vi "Test Panel.vi"(8 "error in (no error)":errorcluster, 11 "Node Ptr":T2 format="%.0x") -> (0 "error out":errorcluster)   [LabVIEW 2019]
uses:
  <vilib>/NI VeriStand/Custom Device API/Custom Device Item Ref.ctl
  <vilib>/NI VeriStand/UI Controls/Tree and Alias Browser/Tree Alias Browser Display.ctl
  NationalInstruments.VeriStand.SystemDefinitionAPI
  NationalInstruments.VeriStand.SystemStorage
  <vilib>/NI VeriStand/Custom Device API/Custom Device API.lvlib
  <vilib>/NI VeriStand/UI Controls/Tree and Alias Browser/NI_VS UI Tree Alias Browser.lvlib
  Software Multi-Plex System Explorer.lvlib
  NationalInstruments.VeriStand.SystemStorageUI
panel:
  in  "error in (no error) 2":errorcluster
  in  "System Definition":path
  in  "Map Input":bool
  out "Input Path":string
  in  "Tree Browser":T1
  in  "Specific Header":cluster{"Section Name":string}={"Section Name"="Specify Input 1 Channel Source"}
  in  "General Header":cluster{"Section Name":string}={"Section Name"="Software Multi-Plex Channel Input 1 Settings"}
  in  "Description":string
  in  "Name":string
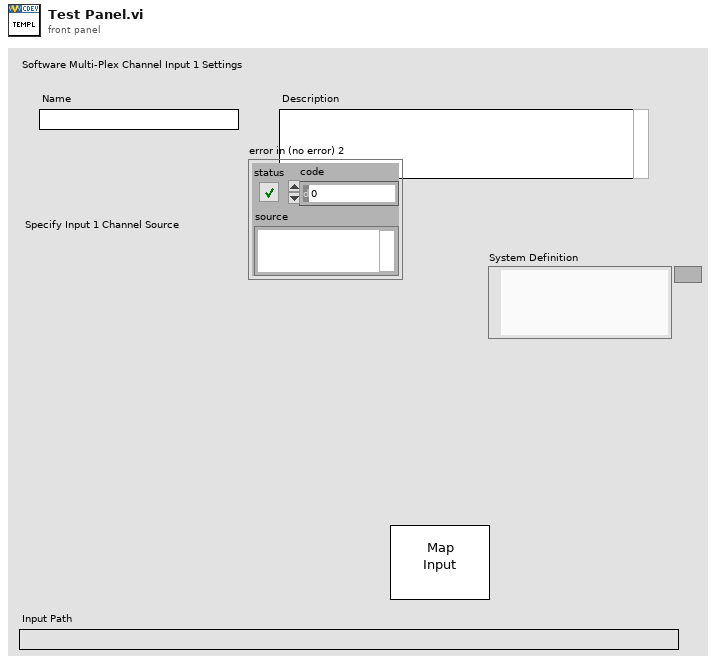
[diagram p1: front panel]
types:
  T1 = typedef "NI_VS UI Tree Alias Browser.lvlib/Tree Alias Browser Display.ctl" = refnum<k24>
  T2 = typedef "Custom Device API.lvlib/Custom Device Item Ref.ctl" = u64
  T3 = typedef "Custom Device API.lvlib/Custom Device Item Info.ctl" = cluster{"Name":string, "Is Channel":bool, "GUID":string, "Is Waveform":bool}
  T4 = typedef "NI_VS UI Tree Alias Browser.lvlib/Callback Type.ctl" = cluster{"Net Callbacks":refnum<k27>[], "Event":T5}
  T5 = typedef "NI_VS UI Tree Alias Browser.lvlib/Net Event Data Ref.ctl" = refnum<user-event>
  T6 = typedef "NI_VS UI Tree Alias Browser.lvlib/Tree Alias Browser Ref.ctl" = refnum<k24>
  T7 = typedef "Custom Device API.lvlib/Custom Device Commands.ctl" = enum16{"Default", "Item renamed", "Shutdown", "Dynamic button pressed"}
  T8 = typedef "NI_VS UI Tree Alias Browser.lvlib/Net Event.ctl" = enum16{"SelectedItem", "DblClick"}
  T9 = typedef "Custom Device API.lvlib/Custom Device Pointer.ctl" = refnum<k24>
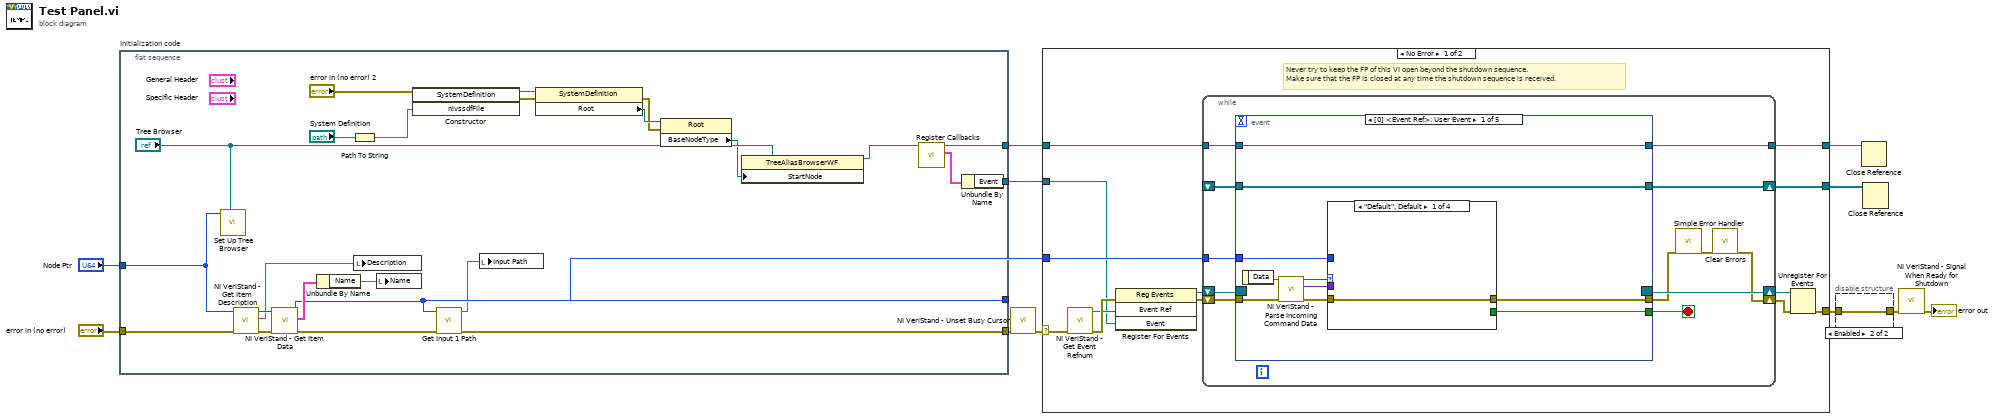
[diagram p0: block diagram]
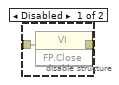
[diagram p2: hidden frame]
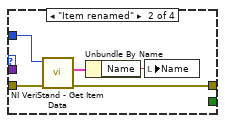
[diagram p3: hidden frame]
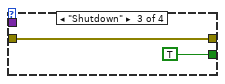
[diagram p4: hidden frame]
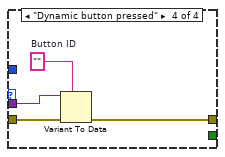
[diagram p5: hidden frame]
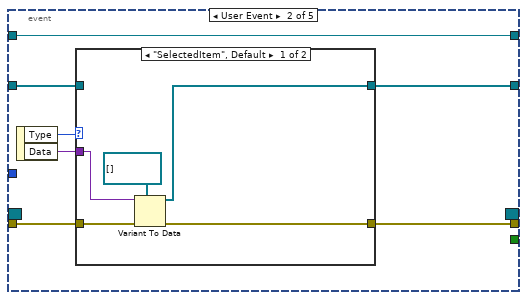
[diagram p6: hidden frame]
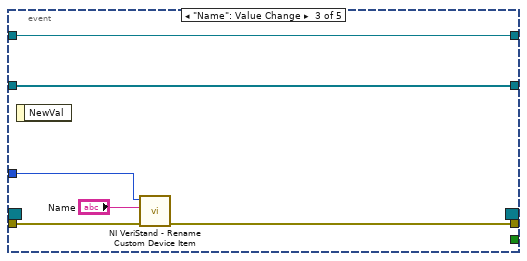
[diagram p8: hidden frame]
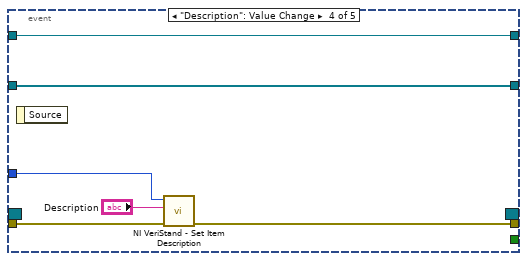
[diagram p9: hidden frame]
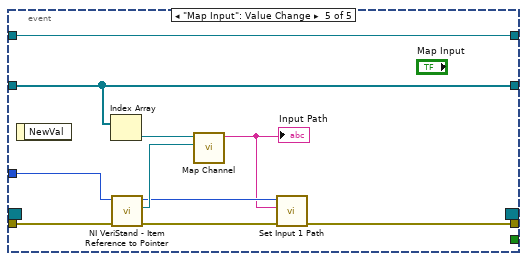
[diagram p10: hidden frame]
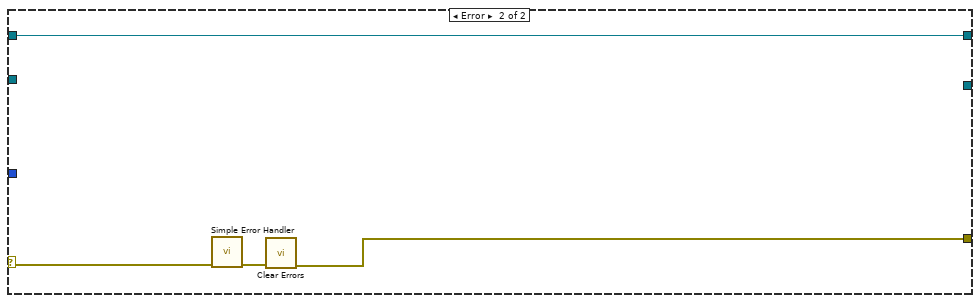
[diagram p11: hidden frame]
diagram:
  n1 = flat-sequence "Initialization code" {
    tunnel: "error in (no error)" -> [w31]
    tunnel: "Node Ptr" -> [w30]
    tunnel: [w25] -> w8
    tunnel: [w24] -> w5
    tunnel: [w29] -> w4
    tunnel: [w27] -> w2
    frame #0 {
      n2 = call "Set Up Tree Browser.vi"("Tree Ref"="Tree Browser", "Item Ref in"=w30) -> ()  [unwired: 10 in]
      n3 = call <vilib>:"NI VeriStand - Get Item Description.vi"("error in (no error)"=w31, "Item Ref in"=w30) -> ("error out"=w35:errorcluster, "Description"=w32:string, "Item Ref out"=w36:T2)  [unwired: 7 out]
      n4 = call <vilib>:"NI VeriStand - Get Item Data.vi"("error in (no error)"=w35, "Item Ref in"=w36) -> ("error out"=w26:errorcluster, "Item Info"=w34:T3, "Item Ref out"=w24:T2)  [unwired: 7 out]
      n5 = Unbundle By Name(w34) -> ("Name"=w33:string)
      n6 = Path To String(path="System Definition") -> (string=w16:string)
      n7 = local write "Description"(w32) -> ()
      n8 = local write "Name"(w33) -> ()
      n9 = constructor class="SystemDefinition"(error in="error in (no error) 2", "nivssdfFile"=w16) -> (reference out=w21:refnum<k24>, error out=w20:errorcluster)  [unwired: 2 in, 2 out]
      n10 = call "Get Input 1 Path.vi"("error in (no error)"=w26, "Item Ref in"=w24) -> ("error out"=w25:errorcluster, "Input Path"=w23:string)  [unwired: 8 in]
      n11 = local write "Input Path"(w23) -> ()
      n12 = property class="SystemDefinition"(reference=w21, error in=w20) -> (error out=w18:errorcluster, "Root"=w19:refnum<k24>)  [unwired: 1 out]
      n13 = property class="Root"(reference=w19, error in=w18) -> ("BaseNodeType"=w13:refnum<k24>)  [unwired: 2 out]
      n14 = property class="TreeAliasBrowserWF"(reference="Tree Browser", "StartNode"=w13) -> (reference out=w14:T1)  [unwired: 1 in, 1 out]
      n15 = call <vilib>:"Register Callbacks.vi"("Tree Alias"=w14) -> ("Callbacks"=w28:T4, "Tree Alias dup"=w29:T6)  [unwired: 8 in, 1 out]
      n16 = Unbundle By Name(w28) -> ("Event"=w27:T5)
    }
  }
  n17 = call <vilib>:"NI VeriStand - Unset Busy Cursor.vi"("error in (no error)"=w8) -> ("error out"=w7:errorcluster)  [unwired: 10 out]
  n18 = case shown="No Error" w7 {
    selector: w7 -> [w41 w123]
    tunnel: [w46 w121] -> w12
    tunnel: w5 -> [w42 _]
    tunnel: w4 -> [w40 w120]
    tunnel: [w39 w120] -> w3
    tunnel: w2 -> [w38 _]
    tunnel: [w37 _] -> w1
    frame No Error {
      # "Never try to keep the FP of this VI open beyond the shutdown sequence.\nMake sure that the FP is closed at any time the shutdown sequence is received."
      n19 = call <vilib>:"NI VeriStand - Get Event Refnum.vi"("error in (no error)"=w41) -> ("error out"=w49:errorcluster, "Event Ref"=w45:refnum<user-event>)  [unwired: 9 out]
      n20 = register-events(error in=w49, w45, w38) -> (reference out=w43:refnum<event-registration>, error out=w44:errorcluster)  [unwired: 1 in]
      n21 = while {
        tunnel: w42 -> [w57]
        shift-right: [w54] -> w47
        shift-left: w44 -> [w60]
        shift-right: [w61] -> w48
        shift-left: w43 -> [w59]
        tunnel: w40 -> [w53]
        tunnel: [w52] -> w39
        shift-right: [w51] -> w37
        shift-left: _ -> [w50]
        stop <- w58 stop-if-true
        n22 = event shown="[0] <Event Ref>: User Event" {
          selector: w59 -> [_ _ _ _ _]
          dyn-events: [_ _ _ _ _] -> w61
          timeout: _ -> [_ _ _ _ _]
          tunnel: w60 -> [w71 w88 w103 w108 w116]
          tunnel: [w67 _ _ _ _] -> w58
          tunnel: [w66 w87 w102 w107 w110] -> w56
          tunnel: w57 -> [w65 _ w101 w109 w115]
          tunnel: w53 -> [w63 w84 w99 w105 w119]
          tunnel: [w63 w84 w99 w105 w119] -> w52
          tunnel: [w62 w86 w98 w104 w118] -> w51
          tunnel: w50 -> [w62 w85 w98 w104 w118]
          event User Event {
            n23 = event-data() -> ("Data"=w70:string)  [unwired: 1 out]
            n24 = call <vilib>:"NI VeriStand - Parse Incoming Command Data.vi"("error in (no error)"=w71, "Incoming data"=w70) -> ("error out"=w69:errorcluster, "Outgoing data"=w64:variant, "Action"=w68:T7)  [unwired: 7 out]
            n25 = case shown="\"Default\", Default" w68 {
              tunnel: w69 -> [w72 w77 w78 w83]
              tunnel: [_ _ TRUE _] -> w67
              tunnel: [w72 w74 w78 w80] -> w66
              tunnel: w65 -> [_ w76 _ _]
              tunnel: w64 -> [_ _ _ w82]
              frame "Default", Default {
              }
              frame "Item renamed" {
                n26 = call <vilib>:"NI VeriStand - Get Item Data.vi"("error in (no error)"=w77, "Item Ref in"=w76) -> ("error out"=w74:errorcluster, "Item Info"=w75:T3)  [unwired: 8 out]
                n27 = Unbundle By Name(w75) -> ("Name"=w73:string)
                n28 = local write "Name"(w73) -> ()
              }
              frame "Shutdown" {
              }
              frame "Dynamic button pressed" {
                w81 = ""  # Button ID
                n29 = Variant To Data(error in=w83, type=w81, Variant=w82) -> (error out=w80:errorcluster)  [unwired: 1 out]
              }
            }
          }
          event User Event {
            n30 = event-data() -> ("Type"=w90:T8, "Data"=w89:variant)  [unwired: 1 out]
            n31 = case shown="\"SelectedItem\", Default" w90 {
              tunnel: w89 -> [w94 _]
              tunnel: w88 -> [w95 w96]
              tunnel: [w92 w96] -> w87
              tunnel: [w91 w97] -> w86
              tunnel: w85 -> [_ w97]
              frame "SelectedItem", Default {
                n32 = Variant To Data(error in=w95, type=refnum<k24>[] [], Variant=w94) -> (data=w91:refnum<k24>[], error out=w92:errorcluster)
              }
              frame "DblClick" {
              }
            }
          }
          event "Name": Value Change {
            n33 = event-data() -> ()  [unwired: 2 out]
            n34 = call <vilib>:"NI VeriStand - Rename Custom Device Item.vi"("error in (no error)"=w103, "New Name"="Name", "Item Ref in"=w101) -> ("error out"=w102:errorcluster)  [unwired: 1 in, 7 out]
          }
          event "Description": Value Change {
            n35 = event-data() -> ()  [unwired: 2 out]
            n36 = call <vilib>:"NI VeriStand - Set Item Description.vi"("error in (no error)"=w108, "Description"="Description", "Item Ref in"=w109) -> ("error out"=w107:errorcluster)  [unwired: 8 out]
          }
          event "Map Input": Value Change {
            n37 = event-data() -> ()  [unwired: 2 out]
            n38 = Index Array(array=w118) -> (element=w117:refnum<k24>)  [unwired: 1 in]
            n39 = call <vilib>:"NI VeriStand - Item Reference to Pointer.vi"("error in (no error)"=w116, "Item Ref in"=w115) -> ("error out"=w113:errorcluster, "Node Pointer"=w114:T9, "Item Ref out"=w112:T2)  [unwired: 6 in, 1 out]
            n40 = call "Map Channel.vi"("Destination"=w114, "Source"=w117) -> ("Source Path"=w111:string)  [unwired: 8 in, 1 out]
            "Input Path" <- w111
            n41 = call "Set Input 1 Path.vi"("error in (no error)"=w113, "Input Path"=w111, "Item Ref in"=w112) -> ("error out"=w110:errorcluster)  [unwired: 8 in]
          }
        }
        n42 = call <vilib>:"Simple Error Handler.vi"("error in (no error)"=w56) -> ("error out"=w55:errorcluster)  [unwired: 1 in, 7 out]
        n43 = call <vilib>:"Clear Errors.vi"("error in (no error)"=w55) -> ("error out"=w54:errorcluster)  [unwired: 1 in, 5 out]
      }
      n44 = Unregister For Events(event registration refnum=w48, error in=w47) -> (error out=w46:errorcluster)
    }
    frame Error {
      n45 = call <vilib>:"Simple Error Handler.vi"("error in (no error)"=w123) -> ("error out"=w122:errorcluster)  [unwired: 1 in, 7 out]
      n46 = call <vilib>:"Clear Errors.vi"("error in (no error)"=w122) -> ("error out"=w121:errorcluster)  [unwired: 1 in, 5 out]
    }
  }
  n47 = disable-structure shown="Enabled" {
    disable-tunnel: w12 -> [w125 w126]
    disable-tunnel: [w124 w126] -> w11
    frame Disabled {
      n48 = invoke class="VI" method="FP.Close"(error in=w125) -> (error out=w124:errorcluster)  [unwired: 2 in, 2 out]
    }
    frame Enabled {
    }
  }
  n49 = Close Reference(reference=w3) -> ()  [unwired: 1 in, 1 out]
  n50 = Close Reference(reference=w1) -> ()  [unwired: 1 in, 1 out]
  n51 = call <vilib>:"NI VeriStand - Signal When Ready for Shutdown.vi"("error in (no error)"=w11) -> ("error out"=→"error out":errorcluster)  [unwired: 10 out]
